vi "die.vi"(6 "timeout in ms (-1)":i32=-1, 7 "references":T1, 8 "error in (no error)":errorcluster) -> (0 "error out":errorcluster)   [LabVIEW 2015, in "lv-recipe-machine.lvlib"]
doc: "This VI will enqueue a command to the input queue which will cause the main loop to stop. It will also write a true to the stop notifier. By default the timeout is -1 (wait forever). In the event that a non negative timeout is provided it will output an error if a timeout occurs."
uses:
  lv-recipe-machine.lvlib
  public/_controls/references.ctl
  public/_controls/input.ctl
  public/_controls/input_command.ctl
  public/_controls/output.ctl
  public/_controls/data.ctl
  public/_controls/configuration.ctl
  public/_controls/recipe_data.ctl
  public/_controls/mode.ctl
  public/_controls/manual_state.ctl
  public/_controls/automatic_state.ctl
  public/_controls/recipe_step.ctl
  <userlib>/antonio-alexander/lv-waitgroup/public/_controls/api_waitgroup.ctl
  public/_controls/change.ctl
  public/_controls/status.ctl
  public/_controls/error.ctl
  <userlib>/antonio-alexander/lv-waitgroup/lv-waitgroup.lvlib
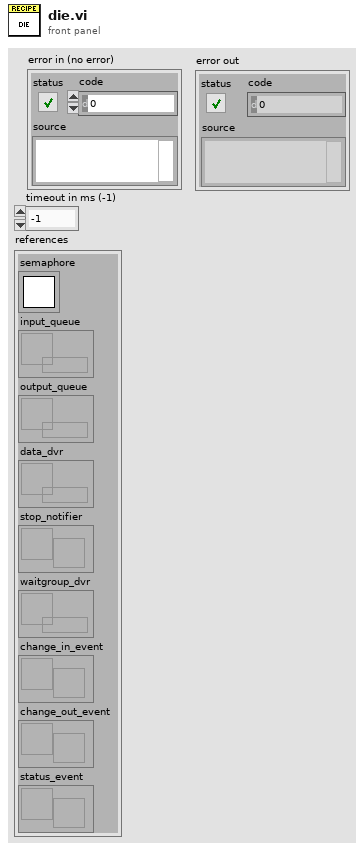
[diagram p1: front panel]
types:
  T1 = typedef "lv-recipe-machine.lvlib/references.ctl" = cluster{"semaphore":T2, "input_queue":refnum<queue>, "output_queue":refnum<queue>, "data_dvr":refnum<data-value>, "stop_notifier":refnum<notifier>, "waitgroup_dvr":refnum<data-value>, "change_in_event":refnum<user-event>, "change_out_event":refnum<user-event>, "status_event":refnum<user-event>}
  T2 = typedef "Semaphore RefNum" = refnum<k1>
  T3 = typedef "lv-recipe-machine.lvlib/input.ctl" = cluster{"command":T4, "data":variant}
  T4 = typedef "lv-recipe-machine.lvlib/input_command.ctl" = enum8{"<input_command>", "die", "<null>"}
  T5 = typedef "lv-recipe-machine.lvlib/error.ctl" = enum16{"<error>", "bad_command", "command_queue_timeout", "stop_notifier_timeout", "die_command_timeout", "not_in_manual_mode", "not_in_automatic_mode", "not_in_automatic_idle", "not_in_automatic_running", "not_in_automatic_paused", "automatic_step_not_found", "manual_step_not_found", "<null>"}
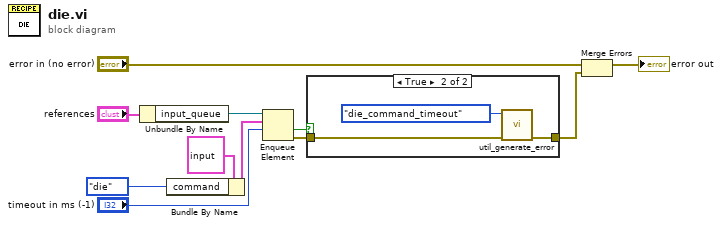
[diagram p0: block diagram]
diagram:
  n1 = Unbundle By Name("references") -> ("input_queue"=w11:refnum<queue>)
  n2 = Bundle By Name(cluster=T3 {"command"=enum."<input_command>", "data"=variant(cluster{"data":variant} {"data"=variant})} ("input"), "command"=input_command."die") -> (w1:T3)
  n3 = Enqueue Element(queue=w11, element=w1, timeout in ms (-1)="timeout in ms (-1)") -> (timed out?=w4:bool, error out=w6:errorcluster)  [unwired: 1 in, 1 out]
  n4 = case shown="True" w4 {
    tunnel: w6 -> [w12 w14]
    tunnel: [w12 w13] -> w5
    frame False {
    }
    frame True {
      n5 = call "util_generate_error.vi"("error in (no error)"=w14, "error"=error."die_command_timeout") -> ("error out"=w13:errorcluster)  [unwired: 9 in]
    }
  }
  n6 = Merge Errors("error in (no error)", w5) -> (→"error out":errorcluster)
